vi "Calculate Window Bounds Error.vi"(11 "Window Bounds":T1) -> (3 "Error (%)":dbl)   [LabVIEW 2020, in "Peer Review.lvclass"]
uses:
  Peer Review.lvclass
  <vilib>/Utility/miscctls.llb/LVRectTypeDef.ctl
  Peer Review.lvclass/Peer Review.ctl
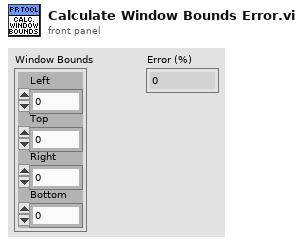
[diagram p1: front panel]
types:
  T1 = typedef "LVRectTypeDef.ctl" = cluster{"Left":i16, "Top":i16, "Right":i16, "Bottom":i16}
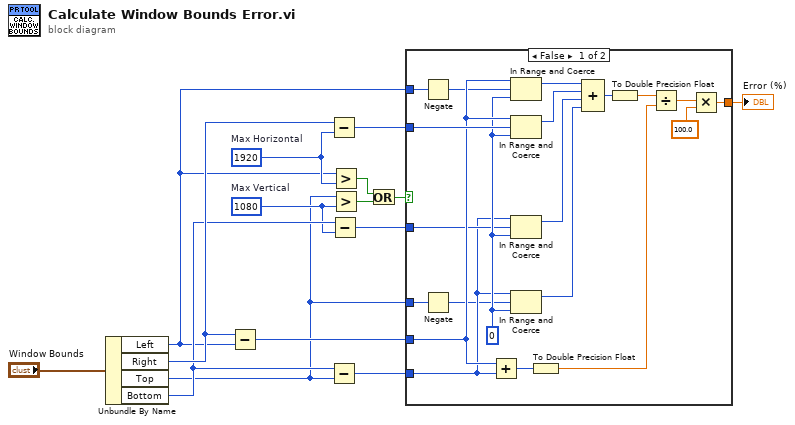
[diagram p0: block diagram]
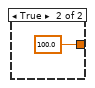
[diagram p2: hidden frame]
diagram:
  w6 = i16 1080  # Max Vertical
  w8 = i16 1920  # Max Horizontal
  n1 = Unbundle By Name("Window Bounds") -> ("Left"=w1:i16, "Right"=w13:i16, "Top"=w2:i16, "Bottom"=w7:i16)
  n2 = Subtract(x=w13, y=w1) -> (x-y=w11:i16)
  n3 = Subtract(x=w13, y=w8) -> (x-y=w12:i16)
  n4 = Subtract(x=w7, y=w2) -> (x-y=w9:i16)
  n5 = Subtract(x=w7, y=w6) -> (x-y=w10:i16)
  n6 = Greater?(x=w1, y=w8) -> (0:w5:bool)
  n7 = Greater?(x=w2, y=w6) -> (0:w4:bool)
  n8 = Or(x=w5, y=w4) -> (x .or. y?=w3:bool)
  n9 = case shown="False" w3 {
    tunnel: [w31 100.0] -> w14
    tunnel: w12 -> [w30 _]
    tunnel: w11 -> [w28 _]
    tunnel: w10 -> [w25 _]
    tunnel: w9 -> [w24 _]
    tunnel: w2 -> [w19 _]
    tunnel: w1 -> [w17 _]
    frame False {
      w26 = i16 0 ("y")
      n10 = Negate(x=w17) -> (-x=w16:i16)
      n11 = Negate(x=w19) -> (-x=w18:i16)
      n12 = Add(x=w28, y=w24) -> (x+y=w34:i16)
      n13 = In Range and Coerce(upper limit=w28, x=w16, lower limit=w26) -> (coerced(x)=w27:i16)  [unwired: 1 out]
      n14 = In Range and Coerce(upper limit=w28, x=w30, lower limit=w26) -> (coerced(x)=w29:i16)  [unwired: 1 out]
      n15 = In Range and Coerce(upper limit=w24, x=w25, lower limit=w26) -> (coerced(x)=w23:i16)  [unwired: 1 out]
      n16 = In Range and Coerce(upper limit=w24, x=w18, lower limit=w26) -> (coerced(x)=w20:i16)  [unwired: 1 out]
      n17 = To Double Precision Float(number=w34) -> (double precision float=w21:dbl)
      n18 = Compound Arithmetic op=ADD(w27, w29, w23, w20) -> (w35:i16)
      n19 = To Double Precision Float(number=w35) -> (double precision float=w22:dbl)
      n20 = Divide(x=w22, y=w21) -> (x/y=w33:dbl)
      n21 = Multiply(x=w33, y=100.0) -> (x*y=w31:dbl)
    }
    frame True {
    }
  }
  "Error (%)" <- w14
